vi "subBuildSpecAndReplaceLibrary.vi"(8 "error in (no error)":errorcluster, 9 "Build spec refs":map{string, refnum<vi>}(c390), 10 "FileInfo":T1, 11 "VI in":refnum<vi>) -> (0 "error out":errorcluster, 1 "Loose files":path[](array[path]), 2 "Result":string, 3 "Message":string)   [LabVIEW 2020, in "SolutionBuilder.lvlib"]
uses:
  SolutionBuilder.lvlib
  FileInfo.ctl
  <vilib>/Utility/miscctls.llb/LVReplaceWithSaveOptionEnum.ctl
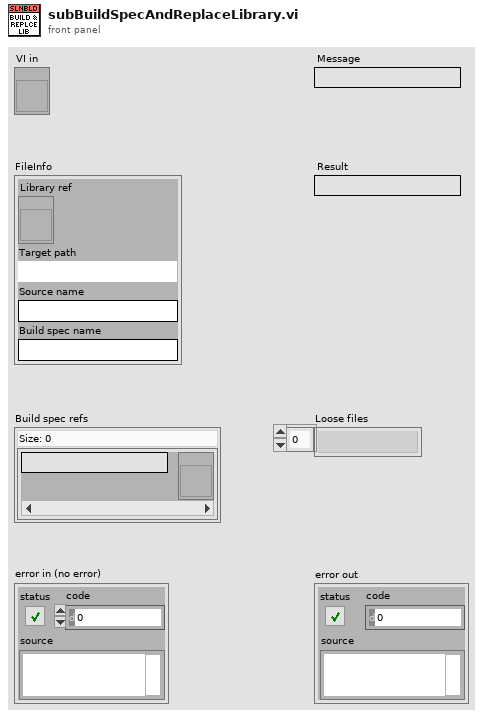
[diagram p1: front panel]
types:
  T1 = typedef "SolutionBuilder.lvlib/FileInfo.ctl" = cluster{"Library ref":refnum<vi>, "Target path":path, "Source name":string, "Build spec name":string}
  T2 = typedef "LVReplaceWithSaveOptionEnum.ctl" = enum16{"Save All Without Prompts", "Save All With Prompts", "Do Not Save (Retain In Memory)"}
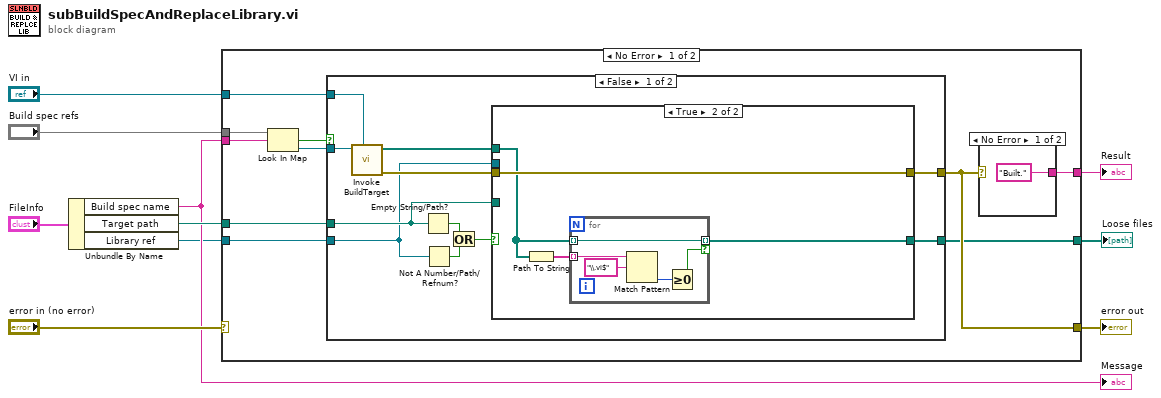
[diagram p0: block diagram]
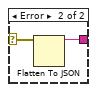
[diagram p2: hidden frame]
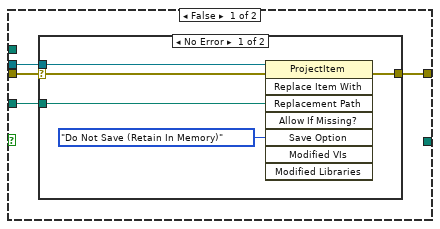
[diagram p3: hidden frame]
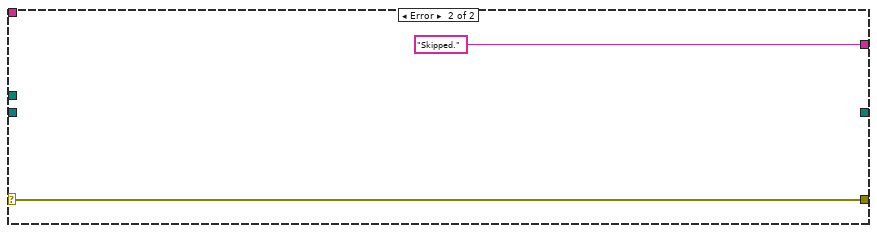
[diagram p6: hidden frame]
diagram:
  n1 = Unbundle By Name("FileInfo") -> ("Build spec name"=w3:string, "Target path"=w9:path, "Library ref"=w2:refnum<vi>)
  "Message" <- w3
  n2 = case shown="No Error" "error in (no error)" {
    selector: "error in (no error)" -> [_ w54]
    tunnel: "VI in" -> [w20 _]
    tunnel: w9 -> [w19 _]
    tunnel: w2 -> [w18 _]
    tunnel: "Build spec refs" -> [w16 _]
    tunnel: w3 -> [w15 _]
    tunnel: [w13 "Skipped." ("JSON string")] -> w6
    tunnel: [w12 w54] -> w4
    tunnel: [w11 _] -> w1
    frame No Error {
      n3 = Look In Map(map=w16, key=w15) -> (key not found?=w14:bool, value=w17:refnum<vi>)  [unwired: 1 in]
      n4 = case shown="False" w14 {
        tunnel: w20 -> [w34 _]
        tunnel: w19 -> [w30 _]
        tunnel: w18 -> [w29 _]
        tunnel: [w33 _] -> w12
        tunnel: w17 -> [w31 _]
        tunnel: [w24 _] -> w11
        frame False {
          n5 = call <vilib>:"Invoke BuildTarget.vi"("vi reference"=w34, "BuildItem ref"=w31) -> ("error out"=w32:errorcluster, "Generated files"=w25:path[])  [unwired: 8 in]
          n6 = Empty String/Path?(string/path=w30) -> (empty?=w28:bool)
          n7 = Not A Number/Path/Refnum?(number/path/refnum=w29) -> (NaN/Path/Refnum?=w27:bool)
          n8 = Or(x=w28, y=w27) -> (x .or. y?=w26:bool)
          n9 = case shown="True" w26 {
            tunnel: w30 -> [w38 _]
            tunnel: w29 -> [w37 _]
            tunnel: [w36 w48] -> w33
            tunnel: w32 -> [w35 w48]
            tunnel: w25 -> [_ w47]
            tunnel: [_ w45] -> w24
            frame False {
              n10 = case shown="No Error" w35 {
                selector: w35 -> [w43 w44]
                tunnel: [w39 w44] -> w36
                tunnel: w37 -> [w42 _]
                tunnel: w38 -> [w40 _]
                frame No Error {
                  n11 = invoke class="ProjectItem" method="Replace Item With"(reference=w42, error in=w43, "Replacement Path"=w40, "Save Option"=LVReplaceWithSaveOptionEnum."Do Not Save (Retain In Memory)") -> (error out=w39:errorcluster)  [unwired: 4 in, 7 out]
                }
                frame Error {
                }
              }
            }
            frame True {
              n12 = Path To String(path=w47) -> (string=w46:string[])
              n13 = for {
                tunnel: w47 -> [w50] mode=indexing
                tunnel: w46 -> [w53] mode=indexing
                tunnel: [w50] -> w45 mode=indexing if=w49
                n14 = Match Pattern(string=w53, regular expression="\\.vi$") -> (offset past match=w51:i32)  [unwired: 1 in, 3 out]
                n15 = Greater Or Equal To 0?(x=w51) -> (x >= 0?=w49:bool)
              }
            }
          }
        }
        frame True {
        }
      }
      n16 = case shown="No Error" w12 {
        selector: w12 -> [_ w23]
        tunnel: ["Built." ("f") w22] -> w13
        frame No Error {
        }
        frame Error {
          n17 = Flatten To JSON(anything=w23) -> (JSON string=w22:string)  [unwired: 2 in, 1 out]
        }
      }
    }
    frame Error {
    }
  }
  "Result" <- w6
  "error out" <- w4
  "Loose files" <- w1
